vi "writeSaveImagesXML.vi"(8 "error in (no error)":errorcluster, 10 "NativeXML in":refnum<class "NativeXML.lvclass">, 11 "WinX32Settings in":refnum<class "WinX32Settings.lvclass">) -> (0 "error out":errorcluster, 2 "NativeXML out":refnum<class "NativeXML.lvclass">, 3 "WinX32Settings out":refnum<class "WinX32Settings.lvclass">)   [LabVIEW 2011, in "Tools.lvlib" / "Settings.lvlib" / "WinX32Settings.lvclass"]
uses:
  WinX32Settings.lvclass
  NativeXML/NativeXML.lvclass
  CamaraSettings.lvclass
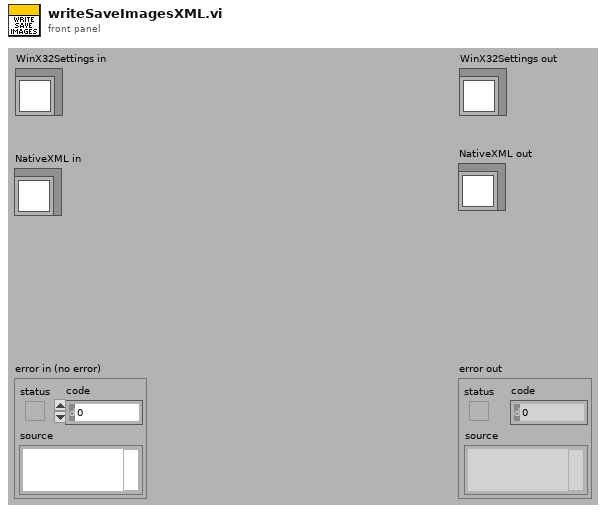
[diagram p1: front panel]
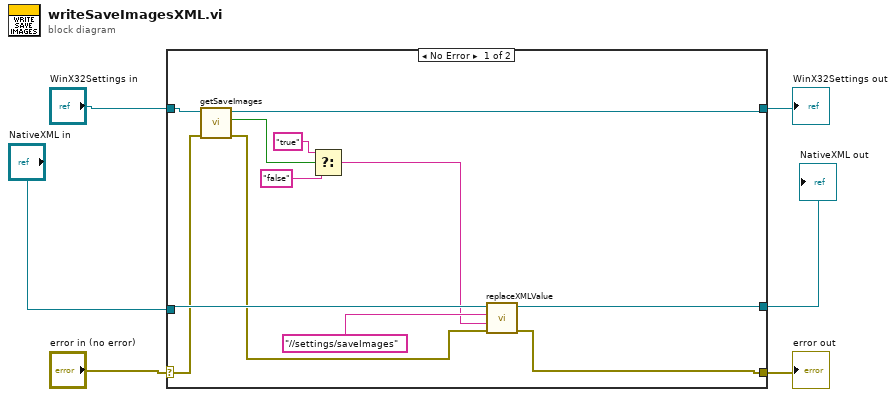
[diagram p0: block diagram]
diagram:
  n1 = case shown="No Error" "error in (no error)" {
    selector: "error in (no error)" -> [w13 w21]
    tunnel: [w15 w21] -> w1
    tunnel: [w7 w20] -> w2
    tunnel: "WinX32Settings in" -> [w14 w20]
    tunnel: "NativeXML in" -> [w18 w19]
    tunnel: [w17 w19] -> w3
    frame No Error {
      n2 = call "getSaveImages.vi"("error in (no error)"=w13, "CamaraSettings in"=w14) -> ("error out"=w12:errorcluster, "saveImages"=w11:bool, "CamaraSettings out"=w7:refnum<class "WinX32Settings.lvclass">)  [unwired: 7 in]
      n3 = Select(t="true", s=w11, f="false") -> (s? t:f=w10:string)
      n4 = call "replaceXMLValue.vi"("error in (no error)"=w12, "value"=w10, "replace in"="//settings/saveImages", "NativeXML in"=w18) -> ("error out"=w15:errorcluster, "NativeXML out"=w17:refnum<class "NativeXML.lvclass">)  [unwired: 6 in]
    }
    frame Error {
    }
  }
  "error out" <- w1
  "WinX32Settings out" <- w2
  "NativeXML out" <- w3
